vi "To Pretty String.vi"(8 "error in (no error)":errorcluster, 11 "JSON Basic Type in":refnum<class "JSON Basic Type.lvclass">) -> (0 "error out":errorcluster, 3 "Pretty Print String":string)   [LabVIEW 2015, in "LVJSON.lvlib" / "JSON Basic Type.lvclass"]
uses:
  JSON Basic Type.lvclass
  LVJSON.lvlib
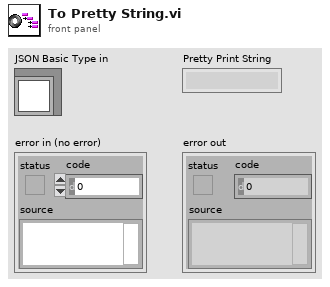
[diagram p1: front panel]
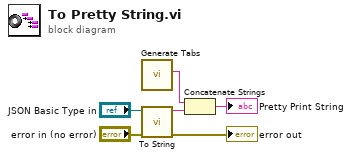
[diagram p0: block diagram]
diagram:
  n1 = call "Generate Tabs.vi"() -> ("Tabs"=w6:string)  [unwired: 10 in, 1 out]
  n2 = call-dynamic "To String.vi"("error in (no error)"="error in (no error)", "JSON Datatype in"="JSON Basic Type in") -> ("error out"=→"error out":errorcluster, "String"=w5:string)  [unwired: 8 in]
  n3 = Concatenate Strings(w6, w5) -> (→"Pretty Print String":string)
